vi "Write Data.vi"(8 "error in (no error)":errorcluster, 10 "Data":string, 11 "String Request Message in":refnum<class "String Request Message.lvclass">) -> (0 "error out":errorcluster, 3 "String Request Message out":refnum<class "String Request Message.lvclass">)   [LabVIEW 2017, in "String Request Message.lvclass"]
uses:
  String Request Message.lvclass
  String Request Message.lvclass/String Request Message.ctl
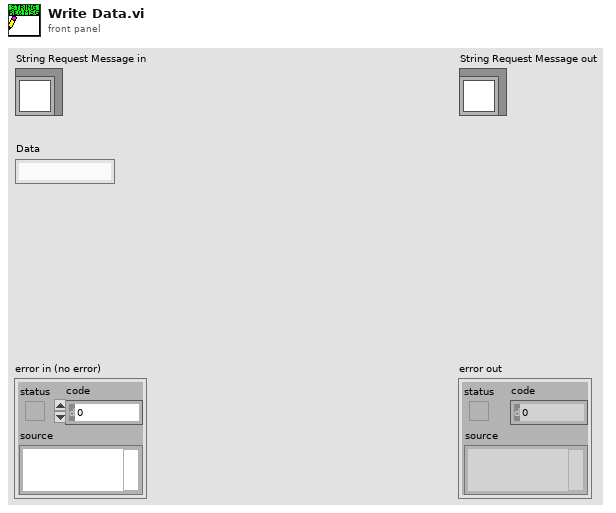
[diagram p1: front panel]
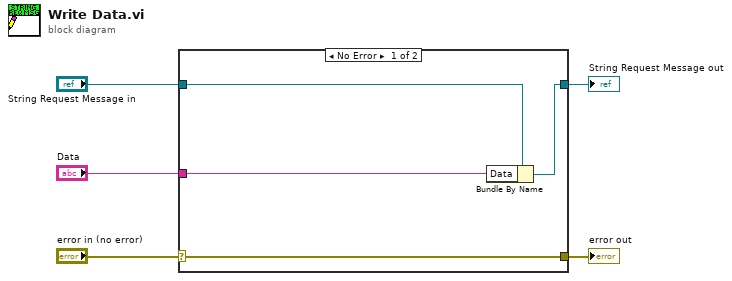
[diagram p0: block diagram]
diagram:
  n1 = case shown="No Error" "error in (no error)" {
    selector: "error in (no error)" -> [w9 w10]
    tunnel: [w9 w10] -> w4
    tunnel: [w7 w11] -> w2
    tunnel: "String Request Message in" -> [w8 w11]
    tunnel: "Data" -> [w6 _]
    frame No Error {
      n2 = Bundle By Name(cluster=w8, "Data"=w6) -> (w7:refnum<class "String Request Message.lvclass">)
    }
    frame Error {
    }
  }
  "error out" <- w4
  "String Request Message out" <- w2
